vi "Network-Create Discovery Events.vi"() -> (8 "Discovery Events":T1)   [LabVIEW 2020]
uses:
  Typedefs/Network-Discovery Events.ctl
  Typedefs/Network-Discovered Host.ctl
  Typedefs/Network-Server Beacon.ctl
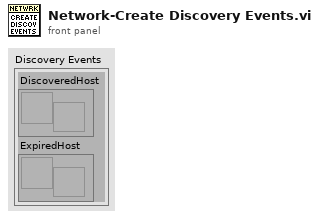
[diagram p1: front panel]
types:
  T1 = typedef "Network-Discovery Events.ctl" = cluster{"DiscoveredHost":refnum<user-event>, "ExpiredHost":refnum<user-event>}
  T2 = typedef "Network-Discovered Host.ctl" = cluster{"Beacon":T3, "Last Seen":timestamp}
  T3 = typedef "Network-Server Beacon.ctl" = cluster{"name":string, "addr":string, "port":u16, "ver":u16}
  T4 = cluster{"DiscoveredHost":refnum<user-event>, "ExpiredHost":refnum<user-event>}
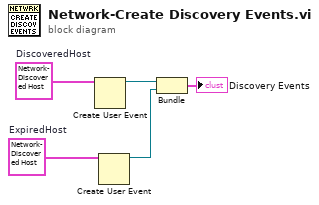
[diagram p0: block diagram]
diagram:
  w4 = T2 {"Beacon"={"name"="", "addr"="", "port"=0, "ver"=10001}, "Last Seen"=timestamp(0 s since 1904-01-01)}  # ExpiredHost
  w5 = T2 {"Beacon"={"name"="", "addr"="", "port"=0, "ver"=10001}, "Last Seen"=timestamp(0 s since 1904-01-01)}  # DiscoveredHost
  n1 = Create User Event(user event datatype=w5) -> (user event=w3:refnum<user-event>)  [unwired: 1 in, 1 out]
  n2 = Create User Event(user event datatype=w4) -> (user event=w2:refnum<user-event>)  [unwired: 1 in, 1 out]
  n3 = Bundle("DiscoveredHost"=w3, "ExpiredHost"=w2) -> (→"Discovery Events":T4)  [unwired: 1 in]
